vi "settings_notifier.vi"() -> (0 "error out":errorcluster, 3 "GLOBAL SETTINGS":refnum<notifier>)   [LabVIEW 2013]
uses:
  main_machine/type_defs/global_settings.ctl
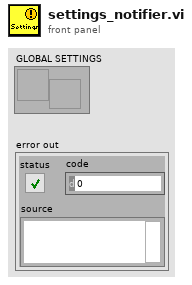
[diagram p1: front panel]
types:
  T1 = typedef "global_settings.ctl" = cluster{"# REACTORS":u32, "17X PORT":i32, "WASTE POSITION ":i32, "SECONDS BETWEEN SAMPLING":dbl, "FACS DIVA DIRECTORY":path, "DATA FILE":path, "REACTORS TO USE":u32[], "PULSE PERIOD":i32, "USE LIGHTS?":bool, "LED FILE":path, "LED CHANNELS":u32[], "PULSE LENGTH":i32, "SUMMARY FILE":path, "OUTGROWTH TIME POINTS":dbl, "SELECTION VALVE PORT":refnum<visa-resource-name>, "HTS PORT":refnum<visa-resource-name>, "DILUTION VOLUME (uL)":i32, "DILUTION FILE":path, "1X PORT":i32}
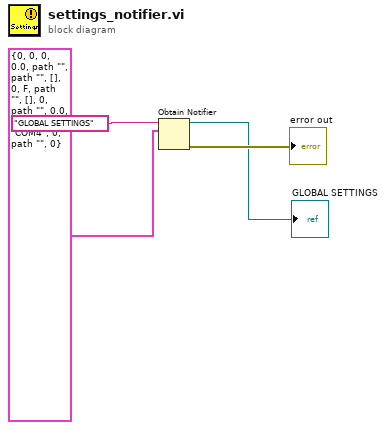
[diagram p0: block diagram]
diagram:
  n1 = Obtain Notifier(name (unnamed)="GLOBAL SETTINGS", notification data type=T1 {"# REACTORS"=0, "17X PORT"=0, "WASTE POSITION "=0, "SECONDS BETWEEN SAMPLING"=0.0, "FACS DIVA DIRECTORY"=path "", "DATA FILE"=path "", "REACTORS TO USE"=[], "PULSE PERIOD"=0, "USE LIGHTS?"=FALSE, "LED FILE"=path "", "LED CHANNELS"=[], "PULSE LENGTH"=0, "SUMMARY FILE"=path "", "OUTGROWTH TIME POINTS"=0.0, "SELECTION VALVE PORT"="COM5", "HTS PORT"="COM4", "DILUTION VOLUME (uL)"=0, "DILUTION FILE"=path "", "1X PORT"=0} ("SETTINGS")) -> (notifier out=→"GLOBAL SETTINGS":refnum<notifier>, error out=→"error out":errorcluster)  [unwired: 2 in, 1 out]
